vi "GetAttachedTaikoSerials.vi"(8 "error in (no error)":errorcluster) -> (2 "Array 2":i32[](array[numeric]), 3 "Array":string[](array[string]))   [LabVIEW 2010]
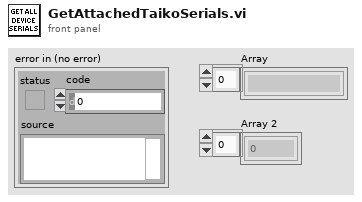
[diagram p1: front panel]
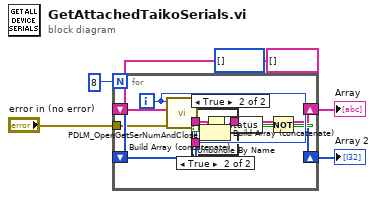
[diagram p0: block diagram]
diagram:
  n1 = for {
    N: 8 -> [_]
    tunnel: "error in (no error)" -> [w15]
    shift-right: [w9] -> w6
    shift-left: string[] [] ("Array 3") -> [w10]
    shift-right: [w7] -> w5
    shift-left: i32[] [] ("Array 3") -> [w8]
    i -> [w14]
    n2 = call "PDLM_OpenGetSerNumAndClose.vi"("error in (no error)"=w15, "USBIdx"=w14) -> ("error out"=w11:errorcluster, "SerNo"=w16:string)  [unwired: 7 in, 1 out]
    n3 = Unbundle By Name(w11) -> ("status"=w13:bool)
    n4 = Not(x=w13) -> (.not. x?=w12:bool)
    n5 = case shown="True" w12 {
      tunnel: w8 -> [w17 w19]
      tunnel: w14 -> [_ w18]
      tunnel: [w17 w20] -> w7
      frame False {
      }
      frame True {
        n6 = Build Array (concatenate)(w19, w18) -> (w20:i32[])
      }
    }
    n7 = case shown="True" w12 {
      tunnel: w10 -> [w21 w23]
      tunnel: w16 -> [_ w22]
      tunnel: [w21 w24] -> w9
      frame False {
      }
      frame True {
        n8 = Build Array (concatenate)(w23, w22) -> (w24:string[])
      }
    }
  }
  "Array" <- w6
  "Array 2" <- w5
